vi "WristDashReadNetwork.vi"() -> (0 "WristGravityCompMotorDmd":dbl, 1 "WristMotorDmd":dbl, 2 "WristPosDeg":dbl, 3 "WristSetpointDeg":dbl, 4 "WristAtSetpoint":bool, 5 "WristProtectHighClampActive":bool, 7 "WristProtectLowClampActive":bool)   [LabVIEW 2023]
uses:
  <vilib>/Rock Robotics/Network Tables/NT Read Number.vi
  <vilib>/Rock Robotics/Network Tables/NT Read Boolean.vi
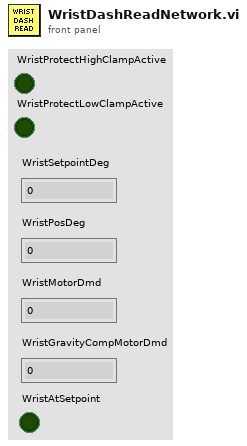
[diagram p1: front panel]
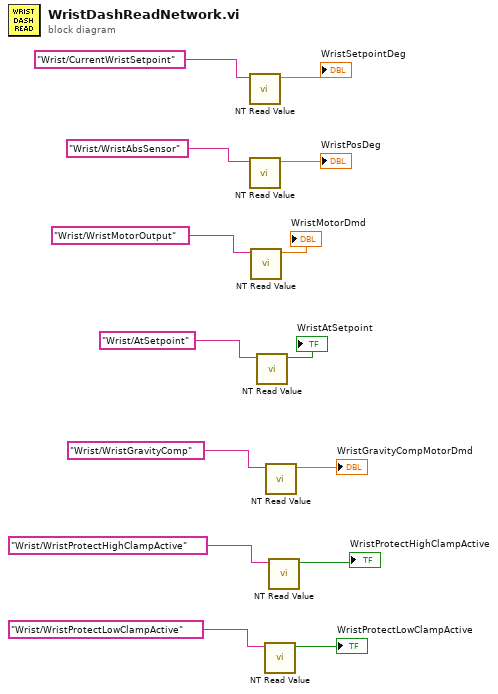
[diagram p0: block diagram]
diagram:
  n1 = call-poly <vilib>:"NT Read Value.vi"("name"="Wrist/CurrentWristSetpoint") -> ("value"=→"WristSetpointDeg":dbl)  [unwired: 8 in, 2 out]
  n2 = call-poly <vilib>:"NT Read Value.vi"("name"="Wrist/WristAbsSensor") -> ("value"=→"WristPosDeg":dbl)  [unwired: 8 in, 2 out]
  n3 = call-poly <vilib>:"NT Read Value.vi"("name"="Wrist/WristMotorOutput") -> ("value"=→"WristMotorDmd":dbl)  [unwired: 8 in, 2 out]
  n4 = call-poly <vilib>:"NT Read Value.vi"("name"="Wrist/AtSetpoint") -> ("value"=→"WristAtSetpoint":bool)  [unwired: 8 in, 2 out]
  n5 = call-poly <vilib>:"NT Read Value.vi"("name"="Wrist/WristProtectLowClampActive") -> ("value"=→"WristProtectLowClampActive":bool)  [unwired: 8 in, 2 out]
  n6 = call-poly <vilib>:"NT Read Value.vi"("name"="Wrist/WristGravityComp") -> ("value"=→"WristGravityCompMotorDmd":dbl)  [unwired: 8 in, 2 out]
  n7 = call-poly <vilib>:"NT Read Value.vi"("name"="Wrist/WristProtectHighClampActive") -> ("value"=→"WristProtectHighClampActive":bool)  [unwired: 8 in, 2 out]
